vi "Save Configuration.vi"(8 "error in":errorcluster, 11 "Module Data":refnum<class "Rename.lvclass">) -> (0 "error out":errorcluster)   [LabVIEW 2015, in "Generic Module Library.lvlib" / "Template G_Module.lvlib"]
uses:
  Template G_Module.lvlib
  <vilib>/Utility/xml.llb/Write to XML File(string).vi
  Module Class/Rename.lvclass
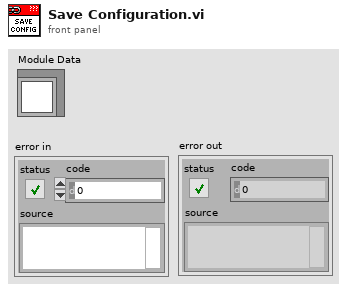
[diagram p1: front panel]
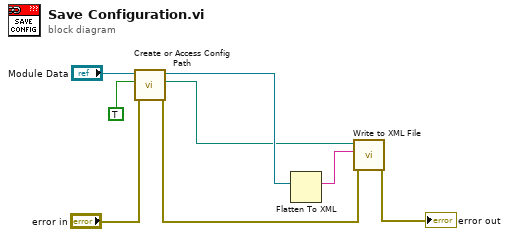
[diagram p0: block diagram]
diagram:
  n1 = call "Create or Access Config Path.vi"("error in"="error in", "Check/Build Folders?"=TRUE, "Module Data"="Module Data") -> ("error out"=w2:errorcluster, "Config File Path"=w4:path, "Module Data"=w5:refnum<class "Rename.lvclass">)  [unwired: 6 in]
  n2 = Flatten To XML(anything=w5) -> (xml string=w3:string)
  n3 = call-poly <vilib>:"Write to XML File.vi"("error in (no error)"=w2, "XML Input"=w3, "XML File Path"=w4) -> ("error out"=→"error out":errorcluster)  [unwired: 6 in, 2 out]
